vi "Set MetaData Priv.vi"(0 "Tree Dict":variant, 5 "Tree ID":string, 7 "MetaData":string, 11 "error in":errorcluster) -> (4 "Tree Dict":variant, 15 "error out":errorcluster)   [LabVIEW 2017, in "Tree API.lvlib" / "Tree.lvclass"]
uses:
  Tree.lvclass
  <vilib>/ErrorRing/Error Ring.xnode
  Typedefs/Tree Cluster.ctl
  <vilib>/Utility/error.llb/Error Cluster From Error Code.vi
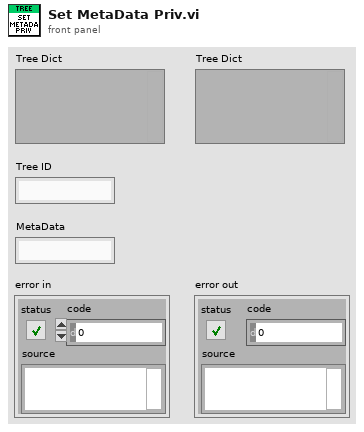
[diagram p1: front panel]
types:
  T1 = typedef "Tree API.lvlib/Tree.lvclass/Tree Cluster.ctl" = cluster{"Unique ID":string, "Parent ID":string, "Child IDs":string[], "Name":string, "MetaData":string, "Data IDs":string[]}
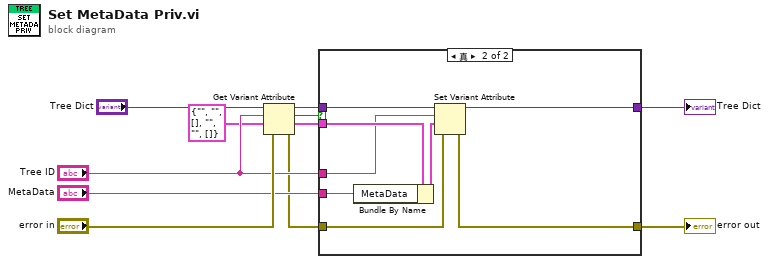
[diagram p0: block diagram]
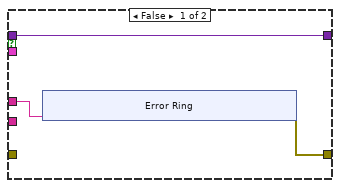
[diagram p2: hidden frame]
diagram:
  n1 = Get Variant Attribute(Variant="Tree Dict", name="Tree ID", default value (empty Variant)=T1 {"Unique ID"="", "Parent ID"="", "Child IDs"=[], "Name"="", "MetaData"="", "Data IDs"=[]} ("Cluster of class private data"), error in="error in") -> (duplicate Variant=w2:variant, found=w4:bool, value=w3:T1, error out=w1:errorcluster)
  n2 = case shown="真" w4 {
    tunnel: w3 -> [_ w25]
    tunnel: w2 -> [w14 w29]
    tunnel: w1 -> [_ w26]
    tunnel: [w13 w27] -> w11
    tunnel: [w14 w28] -> w6
    tunnel: "Tree ID" -> [w12 w23]
    tunnel: "MetaData" -> [_ w22]
    frame False {
      n3 = xnode "Error Ring"("参数 0"=w12) -> ("错误输出"=w13:errorcluster)
    }
    frame True {
      n4 = Bundle By Name(cluster=w25, "MetaData"=w22) -> (w24:T1)
      n5 = Set Variant Attribute(Variant=w29, name=w23, value=w24, error in=w26) -> (Variant out=w28:variant, error out=w27:errorcluster)  [unwired: 1 out]
    }
  }
  "error out" <- w11
  "Tree Dict" <- w6
